vi "Pulse.vi"(3 "Pulse_Durration (ms)":u32=20, 4 "Trigger":bool, 5 "State_In":bool) -> (1 "State_Out":bool)   [LabVIEW 2018]
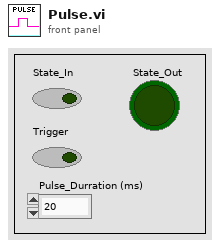
[diagram p1: front panel]
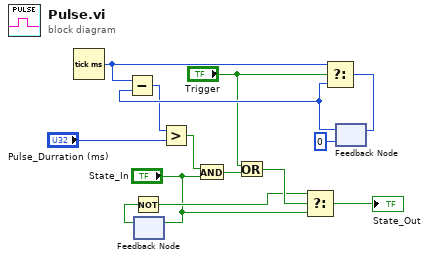
[diagram p0: block diagram]
diagram:
  n1 = Tick Count (ms)() -> (millisecond timer value=w12:u32)
  n2 = feedback-in #1("State_In") -> ()
  n3 = feedback #1() -> (w4:bool)  [unwired: 1 in]
  n4 = Not(x=w4) -> (.not. x?=w3:bool)
  n5 = feedback #2(u32 0 ("millisecond timer value")) -> (w11:u32)
  n6 = Subtract(x=w12, y=w11) -> (x-y=w9:u32)
  n7 = Greater?(x=w9, y="Pulse_Durration (ms)") -> (0:w8:bool)
  n8 = And(x=w8, y="State_In") -> (x .and. y?=w7:bool)
  n9 = Or(x="Trigger", y=w7) -> (x .or. y?=w5:bool)
  n10 = Select(t=w3, s=w5, f="State_In") -> (s? t:f=→"State_Out":bool)
  n11 = Select(t=w12, s="Trigger", f=w11) -> (s? t:f=w14:u32)
  n12 = feedback-in #2(w14) -> ()
